vi "Wrapper_getName_Mod.vi"(8 "error in (no error)":errorcluster caption="entrée d'erreur (pas d'erreur)", 10 "Wrapper":u32, 11 "Index":i32) -> (0 "error out":errorcluster caption="sortie d'erreur", 2 "Spectrometer Name":string)   [LabVIEW 2024]
uses:
  OmniDriver32.dll
  common32.dll
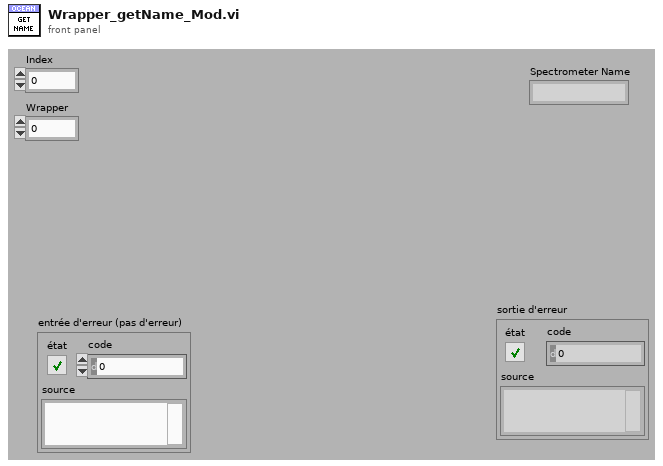
[diagram p1: front panel]
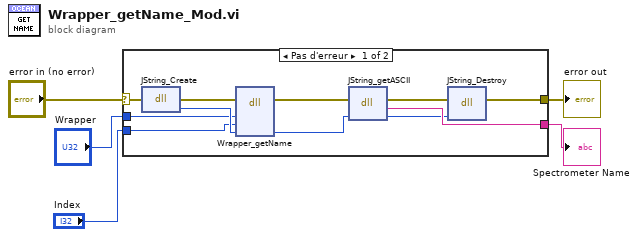
[diagram p0: block diagram]
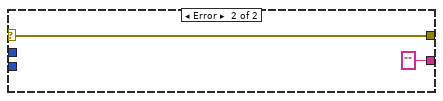
[diagram p2: hidden frame]
diagram:
  n1 = case shown="Pas d'erreur" "error in (no error)" {
    selector: "error in (no error)" -> [w10 w18]
    tunnel: "Index" -> [w15 _]
    tunnel: "Wrapper" -> [w14 _]
    tunnel: [w12 ""] -> w3
    tunnel: [w6 w18] -> w1
    frame No Error {
      n2 = dll-call lib="common32.dll" fn="JString_Create" label="JString.Create"(error in=w10) -> (error out=w9:errorcluster, w16:u32)  [unwired: 2 in, 1 out]
      n3 = dll-call lib="OmniDriver32.dll" fn="Wrapper_getName" label="Wrapper.getName"(error in=w9, "Wrapper"=w14, "Index"=w15, "JString"=w16) -> (error out=w8:errorcluster, "JString"=w13:u32)  [unwired: 5 in, 1 out]
      n4 = dll-call lib="common32.dll" fn="JString_getASCII" label="JString.getASCII"(error in=w8, "JString"=w13) -> (error out=w7:errorcluster, w12:string, "JString"=w11:u32)  [unwired: 2 in, 1 out]
      n5 = dll-call lib="common32.dll" fn="JString_Destroy" label="JString.Destroy"(error in=w7, "JString"=w11) -> (error out=w6:errorcluster)  [unwired: 4 in, 1 out]
    }
    frame Error {
    }
  }
  "Spectrometer Name" <- w3
  "error out" <- w1
